vi "EuniceF_Project2Labview.vi"() -> ()   [LabVIEW 2025]
panel:
  out "System Failure":bool
  out "Low Pressure":bool
  out "P, kPa":dbl(slide) scale=0.0..10.0
  out "P, H20":dbl(slide) scale=0.0..10.0
  out "Isens, mA":dbl(slide) scale=0.0..25.0 scale format="%02.2f"
  out "Vscc, V":dbl(slide) scale=0.0..6.0 scale format="%03.2f"
  out "A to D":i16 format="%x"
  in  "stop":bool
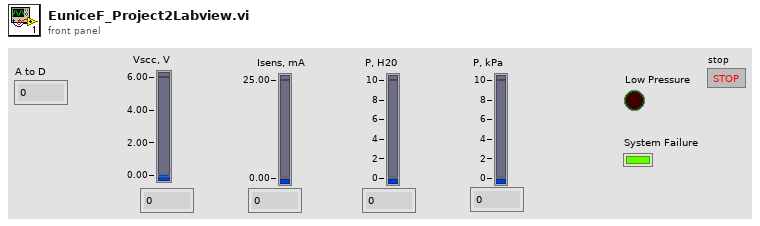
[diagram p1: front panel]
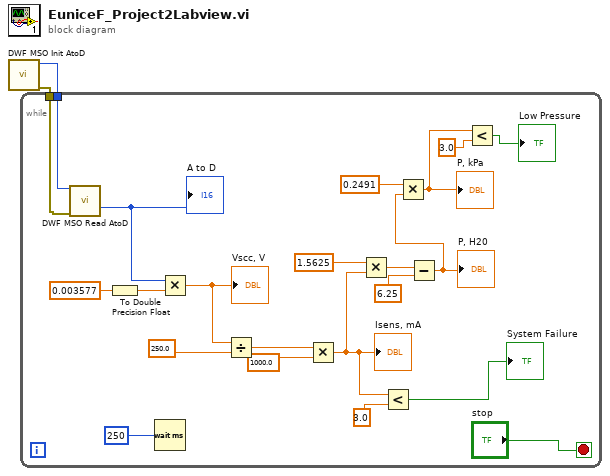
[diagram p0: block diagram]
diagram:
  n1 = call "DWF MSO Init AtoD.vi"() -> ("Error Out"=w1:errorcluster, "Instrument Handle Out"=w2:i32)  [unwired: 10 in]
  n2 = while {
    tunnel: w2 -> [w22]
    tunnel: w1 -> [w21]
    stop <- "stop" stop-if-true
    n3 = call "DWF MSO Read AtoD.vi"("Instrument Handle In AtoD"=w22, "Error In"=w21) -> ("AtoD"=w18:i16)  [unwired: 12 in, 1 out]
    "A to D" <- w18
    n4 = To Double Precision Float(number=0.003577 ("y")) -> (double precision float=w19:dbl)
    n5 = Wait (ms)(milliseconds to wait=u32 250) -> ()  [unwired: 1 out]
    n6 = Multiply(x=w18, y=w19) -> (x*y=w17:dbl)
    "Vscc, V" <- w17
    n7 = Divide(x=w17, y=250.0) -> (x/y=w15:dbl)
    n8 = Multiply(x=w15, y=1000.0) -> (x*y=w3:dbl)
    "Isens, mA" <- w3
    n9 = Multiply(x=1.5625, y=w3) -> (x*y=w12:dbl)
    n10 = Less?(x=w3, y=3.0) -> (x < y?=→"System Failure":bool)
    n11 = Subtract(x=w12, y=6.25) -> (x-y=w9:dbl)
    "P, H20" <- w9
    n12 = Multiply(x=0.2491 ("y"), y=w9) -> (x*y=w6:dbl)
    "P, kPa" <- w6
    n13 = Less?(x=w6, y=3.0) -> (x < y?=→"Low Pressure":bool)
  }
